vi "general setting.vi"() -> ()   [LabVIEW 2019, in "Setting Lib.lvlib"]
uses:
  Setting Lib.lvlib
  database.lvlib
panel:
  in  "Projector Level":i32=10
  out "Error out":errorcluster
  in  "Close":bool
  in  "Projector Check File Path":path
  in  "Processing File Path":path
  in  "Database Refresh Period (day)":i32=30
  in  "Data Saving Period (minute)":i32=10
  out "String":string
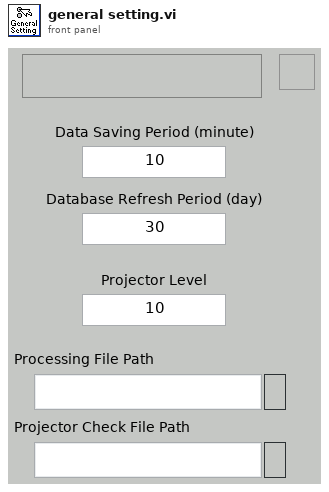
[diagram p1: front panel]
types:
  T1 = enum8{"Enabled", "Disabled", "Disabled and Grayed Out"}
  T2 = cluster{"Data Saving Period (minute)":i32, "Database Refresh Period (day)":i32, "Processing File Path":path, "Projector Check File Path":path}
  T3 = cluster{"Data Saving Period (minute)":i32, "Database Refresh Period (day)":i32, "Processing File Path":path, "Projector Check File Path":path}[]
  T4 = cluster{"Data Saving Period (minute)":i32, "Database Refresh Period (day)":i32, string, string}
  T5 = cluster{i32, "date/time string":string, "date/time string":string, "table":string}
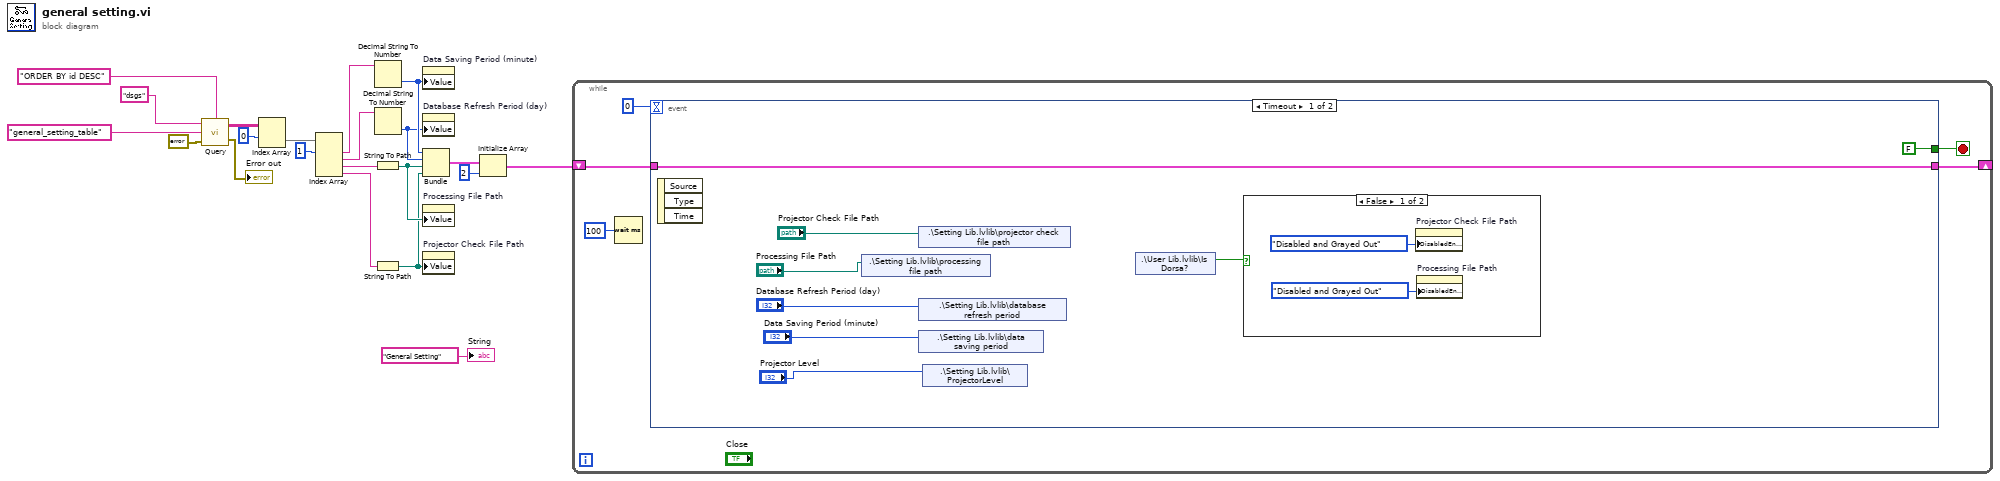
[diagram p0: block diagram]
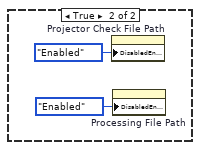
[diagram p2: hidden frame]
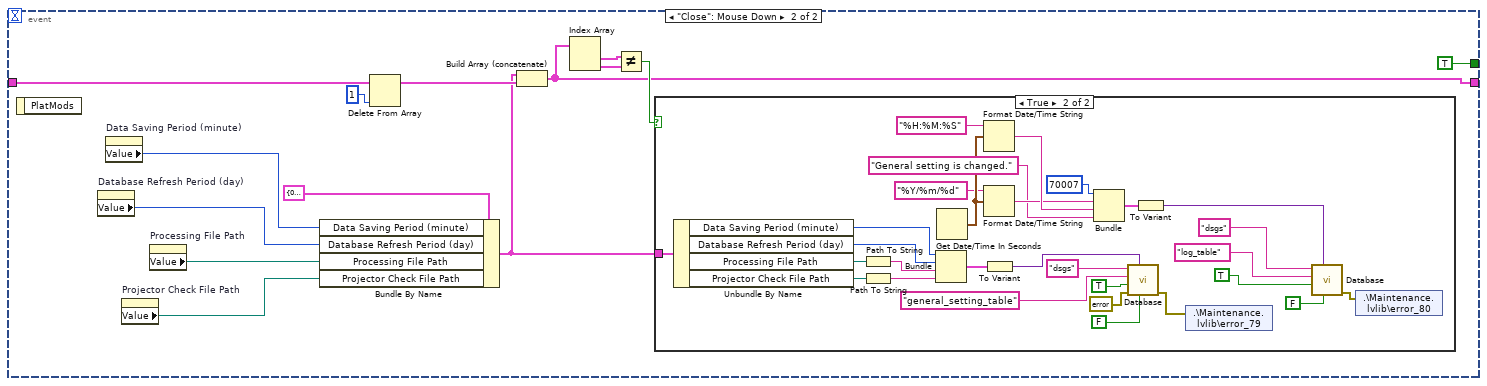
[diagram p3: hidden frame]
diagram:
  n1 = call "Query.vi"("Condition"="ORDER BY id DESC", "Error in"=errorcluster {"status"=FALSE, "code"=0, "source"=""}, "Table Name"="general_setting_table", "Connection Name"="dsgs") -> ("Error out"=→"Error out":errorcluster, "data"=w14:string[][])
  n2 = Index Array(array=w14, index (row)=0) -> (element=w12:string[])  [unwired: 1 in]
  n3 = Index Array(array=w12, index #1=1 ("index")) -> (element #1=w10:string, element #2=w9:string, element #3=w7:string, element #4=w8:string)  [unwired: 3 in]
  n4 = Decimal String To Number(string=w10) -> (number=w6:i32)  [unwired: 2 in, 1 out]
  n5 = Decimal String To Number(string=w9) -> (number=w5:i32)  [unwired: 2 in, 1 out]
  n6 = String To Path(string=w7) -> (path=w4:path)
  n7 = String To Path(string=w8) -> (path=w3:path)
  n8 = property on="Data Saving Period (minute)" class="DigNum (strict)"("Value"=w6) -> ()  [unwired: 2 in, 2 out]
  n9 = property on="Database Refresh Period (day)" class="DigNum (strict)"("Value"=w5) -> ()  [unwired: 2 in, 2 out]
  n10 = Bundle(w6, w5, w4, w3) -> (w2:cluster{i32, i32, path, path})  [unwired: 1 in]
  n11 = property on="Processing File Path" class="Path"("Value"=w4) -> ()  [unwired: 2 in, 2 out]
  n12 = property on="Projector Check File Path" class="Path"("Value"=w3) -> ()  [unwired: 2 in, 2 out]
  n13 = Initialize Array(w2, 2 ("dimension size")) -> (w19:cluster{i32, i32, path, path}[])
  n14 = while {
    shift-right: [w22] -> _
    shift-left: w19 -> [w23]
    stop <- w25 stop-if-true
    n15 = Wait (ms)(milliseconds to wait=u32 100) -> ()  [unwired: 1 out]
    n16 = event shown="[0] Timeout" {
      selector: _ -> [_ _]
      dyn-events: _ -> [_ _]
      timeout: 0 -> [_ _]
      tunnel: [FALSE TRUE] -> w25
      tunnel: w23 -> [w29 w44]
      tunnel: [w29 w43] -> w22
      event Timeout {
        n17 = event-data() -> ()  [unwired: 1 in, 3 out]
        n18 = shared-variable ".\\Setting Lib.lvlib\\processing file path"("Processing File Path") -> ()  [unwired: 1 in, 1 out]
        n19 = shared-variable ".\\Setting Lib.lvlib\\projector check file path"("Projector Check File Path") -> ()  [unwired: 1 in, 1 out]
        n20 = shared-variable ".\\Setting Lib.lvlib\\database refresh period"("Database Refresh Period (day)") -> ()  [unwired: 1 in, 1 out]
        n21 = shared-variable ".\\Setting Lib.lvlib\\data saving period"("Data Saving Period (minute)") -> ()  [unwired: 1 in, 1 out]
        n22 = shared-variable ".\\Setting Lib.lvlib\\ProjectorLevel"("Projector Level") -> ()  [unwired: 1 in, 1 out]
        n23 = shared-variable ".\\User Lib.lvlib\\Is Dorsa?"() -> (w28:bool)  [unwired: 1 in, 1 out]
        n24 = case shown="False" w28 {
          frame False {
            n25 = property on="Projector Check File Path" class="Path"("DisabledEnum"=T1."Disabled and Grayed Out" ("Disabled")) -> ()  [unwired: 2 in, 2 out]
            n26 = property on="Processing File Path" class="Path"("DisabledEnum"=T1."Disabled and Grayed Out" ("Disabled")) -> ()  [unwired: 2 in, 2 out]
          }
          frame True {
            n27 = property on="Projector Check File Path" class="Path"("DisabledEnum"=T1."Enabled" ("Disabled")) -> ()  [unwired: 2 in, 2 out]
            n28 = property on="Processing File Path" class="Path"("DisabledEnum"=T1."Enabled" ("Disabled")) -> ()  [unwired: 2 in, 2 out]
          }
        }
      }
      event "Close": Mouse Down {
        n29 = event-data() -> ()  [unwired: 1 in, 1 out]
        n30 = property on="Database Refresh Period (day)" class="DigNum (strict)"() -> ("Value"=w39:i32)  [unwired: 2 in, 2 out]
        n31 = property on="Data Saving Period (minute)" class="DigNum (strict)"() -> ("Value"=w40:i32)  [unwired: 2 in, 2 out]
        n32 = property on="Projector Check File Path" class="Path"() -> ("Value"=w41:path)  [unwired: 2 in, 2 out]
        n33 = property on="Processing File Path" class="Path"() -> ("Value"=w42:path)  [unwired: 2 in, 2 out]
        n34 = Bundle By Name(cluster=T2 {"Data Saving Period (minute)"=0, "Database Refresh Period (day)"=0, "Processing File Path"=path "", "Projector Check File Path"=path ""}, "Data Saving Period (minute)"=w40, "Database Refresh Period (day)"=w39, "Processing File Path"=w42, "Projector Check File Path"=w41) -> (w47:T2)
        n35 = Delete From Array(array=w44, index=1) -> (array with subset deleted=w51:cluster{i32, i32, path, path}[])  [unwired: 1 in, 1 out]
        n36 = Build Array (concatenate)(w47, w51) -> (w43:T3)
        n37 = Index Array(array=w43) -> (element #1=w50:T2, element #2=w49:T2)  [unwired: 2 in]
        n38 = Not Equal?(x=w50, y=w49) -> (x != y?=w48:bool)
        n39 = case shown="True" w48 {
          tunnel: w47 -> [_ w62]
          frame False {
          }
          frame True {
            n40 = Unbundle By Name(w62) -> ("Data Saving Period (minute)"=w59:i32, "Database Refresh Period (day)"=w58:i32, "Processing File Path"=w60:path, "Projector Check File Path"=w61:path)
            n41 = Path To String(path=w60) -> (string=w57:string)
            n42 = Path To String(path=w61) -> (string=w56:string)
            n43 = Bundle("Data Saving Period (minute)"=w59, "Database Refresh Period (day)"=w58, w57, w56) -> (w55:T4)  [unwired: 1 in]
            n44 = Get Date/Time In Seconds() -> (seconds since 1Jan1904=w77:timestamp)
            n45 = Format Date/Time String(time format string (%c)="%H:%M:%S", seconds (now)=w77) -> (date/time string=w79:string)  [unwired: 1 in]
            n46 = Format Date/Time String(time format string (%c)="%Y/%m/%d", seconds (now)=w77) -> (date/time string=w78:string)  [unwired: 1 in]
            n47 = To Variant(anything=w55) -> (Variant=w63:variant)
            n48 = Bundle(70007, "date/time string"=w78, "date/time string"=w79, "table"="General setting is changed.") -> (w80:T5)  [unwired: 1 in]
            n49 = call "Database.vi"("Delete row?"=FALSE, "Data"=w63, "Error in"=errorcluster {"status"=FALSE, "code"=0, "source"=""}, "Auto Increment ID?"=TRUE, "Table"="general_setting_table", "Connection"="dsgs") -> ("Error out"=w54:errorcluster)  [unwired: 5 in]
            n50 = To Variant(anything=w80) -> (Variant=w81:variant)
            n51 = shared-variable ".\\Maintenance.lvlib\\error_79"(w54) -> ()  [unwired: 1 in, 1 out]
            n52 = call "Database.vi"("Delete row?"=FALSE, "Data"=w81, "Auto Increment ID?"=TRUE, "Table"="log_table" ("table"), "Connection"="dsgs" ("table")) -> ("Error out"=w53:errorcluster)  [unwired: 6 in]
            n53 = shared-variable ".\\Maintenance.lvlib\\error_80"(w53) -> ()  [unwired: 1 in, 1 out]
          }
        }
      }
    }
  }
  "String" <- "General Setting" ("String")
